vi "Acqusition & Generation (Snapshot) test.vi"() -> ()   [LabVIEW 2014]
uses:
  <vilib>/Platform/TimedLoop/XDataNode/timing_clust.ctl
  <vilib>/Platform/TimedLoop/XDataNode/nitl_modes.ctl
  <vilib>/Platform/TimedLoop/XDataNode/wakeup.ctl
  <vilib>/rvi/Emulation/niFpgaSctlEmulationGetInTimedLoop.vi
  <vilib>/rvi/Emulation/niFpgaEmulationReportErrorSimple.vi
  <vilib>/rvi/Emulation/niFpgaGetClockAttributes.vi
  <vilib>/rvi/Emulation/niFpgaCriticalErrorInLSC.vi
  <vilib>/rvi/Emulation/niFpgaEmulationIsFPGAContextNoSignature.vi
  <vilib>/rvi/DataTransferAndStorage/Container/Common/niFpgaContainerGetUniqueNameForEmu.vi
  <vilib>/rvi/Memory/Memory_Emulation/niFpgaMemoryEmulationCacheClearOnFirstRun.vi
  <vilib>/rvi/Memory/Memory_Emulation/nirvimemoryEmulationManagerCache_MakeExclusive.vi
  <vilib>/rvi/Memory/Memory_Emulation/niFpgaMemoryEmulationValidateCache.vi
  <vilib>/rvi/Memory/Memory_Emulation/nirvimemoryEmulationManagerCache_InsertValue.vi
  <vilib>/Utility/error.llb/Clear Errors.vi
  <vilib>/rvi/Memory/Memory_Emulation/nirvimemoryEmulationManagerCache_ReleaseExclusive.vi
  <vilib>/rvi/Memory/Memory_Emulation/nirvimemoryEmulationManagerCache_GetValue.vi
  <vilib>/rvi/Memory/Memory_Emulation/nirvimemoryEmulationManagerCache_SetValue.vi
  <vilib>/rvi/Emulation/niFpgaProcessEmulError.vi
  <vilib>/rvi/errors/niFpgaSetErrorForExecOnDevCompSimple.vi
  <vilib>/rvi/eio/common/nirviEmuReportErrorAndStop.vi
  <vilib>/rvi/FIFO/Fifo_Resource/nirvififoEmulationSetSize.vi
  <vilib>/rvi/FIFO/Fifo_Resource/nirviFifoEmulationQueueMgr.vi
  <instcachedir>/0/nirviFifoEmulationQueueMgr_E5CAEC123FF24DC58D834DCA3CDAA9B5.lvgen/nirviFifoEmulationQueueMgr_E5CAEC123FF24DC58D834DCA3CDAA9B5_010.vi
  <vilib>/rvi/FIFO/Fifo_Resource/nirvififoEmulationDetermineInputValidOut.vi
  <vilib>/rvi/FIFO/Fifo_Resource/nirvififoEmulationCreateLock.vi
  <vilib>/rvi/FIFO/Fifo_Resource/nirvififoEmulationObtainLock.vi
  <vilib>/rvi/FIFO/Fifo_Resource/nirvififoEmulationReleaseLock.vi
  <vilib>/rvi/occurrence/nirviWaitOnOccurrenceBase.vi
  <vilib>/rvi/errors/nirviReportUnexpectedCaseInternalError.vi
  <vilib>/rvi/errors/nirviReportUnexpectedCaseInternalError (U32).vi
  <vilib>/rvi/Memory/Memory_Emulation/nirvimemoryFastEmulation.vi
  <vilib>/rvi/Memory/Memory_Emulation/nirvimemoryEmulation.vi
  <vilib>/rvi/interface/RandomDataEmulation/niFpgaRandomDataHandleErrors.vi
  <vilib>/rvi/eio/common/nirviEmuTemplateMethod_errors.vi
  <vilib>/Platform/TimedLoop/XDataNode/XDataNode.xnode
  <vilib>/rvi/DataTransferAndStorage/Container/XNode/niFpgaContainer.xnode
  <vilib>/rvi/DataTransferAndStorage/Register/Emulation/niFpgaRegisterEmulation.vi
  <vilib>/rvi/FIFO/Fifo_Resource/nirvififoEmulationWrite.vi
  <vilib>/rvi/interface/RandomDataEmulation/nirviRandomDataFpgaReadWriteTemplate.vi
  <vilib>/rvi/FIFO/Fifo_Resource/nirvififoEmulationRead.vi
  <vilib>/eio/EIOMethodNode/EIOMethodNode.xnode
  <vilib>/Platform/TimedLoop/XDataNode/XDNodeRunTimeDep.lvlib
panel:
  in  "Snapshot":bool
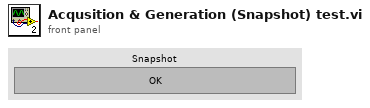
[diagram p1: front panel]
types:
  T1 = typedef "XDNodeRunTimeDep.lvlib/timing_clust.ctl" = cluster{"Expected End [f-1]":u64, "Actual End [f-1]":u64, "Finished Late? [f-1]":bool, "Expected End [i-1]":u64, "Actual End [i-1]":u64, "Finished Late? [i-1]":bool, "Expected Start [i]":u64, "Actual Start [i]":u64, "Expected Start [f]":u64, "Actual Start [f]":u64, "Source Name":string, "Structure Name":string, "Period":i64, "Deadline":i64, "Offset":i64, "Start":i64, "Priority":i32, "Timeout":i32, "Mode":T2, "Wakeup Reason":T3, "Error":errorcluster, "Source Type":string, "Secondary Source Type":string, "Global End Time":u64, "Global Start Time":u64, "Frame Duration":u64, "Iteration Duration":u64, "Assigned CPU":i32, "I/O Scan Engine Mode":u32}
  T2 = typedef "XDNodeRunTimeDep.lvlib/nitl_modes.ctl" = enum32{"No Change", "Process missed periods, maintain original phase", "Discard missed periods, maintain original phase", "Process missed periods, ignore original phase", "Discard missed periods, ignore original phase"}
  T3 = typedef "XDNodeRunTimeDep.lvlib/wakeup.ctl" = enum32{"Normal", "Aborted", "Asynchronous wakeup", "Timing source error", "Timed loop error", "Timeout"}
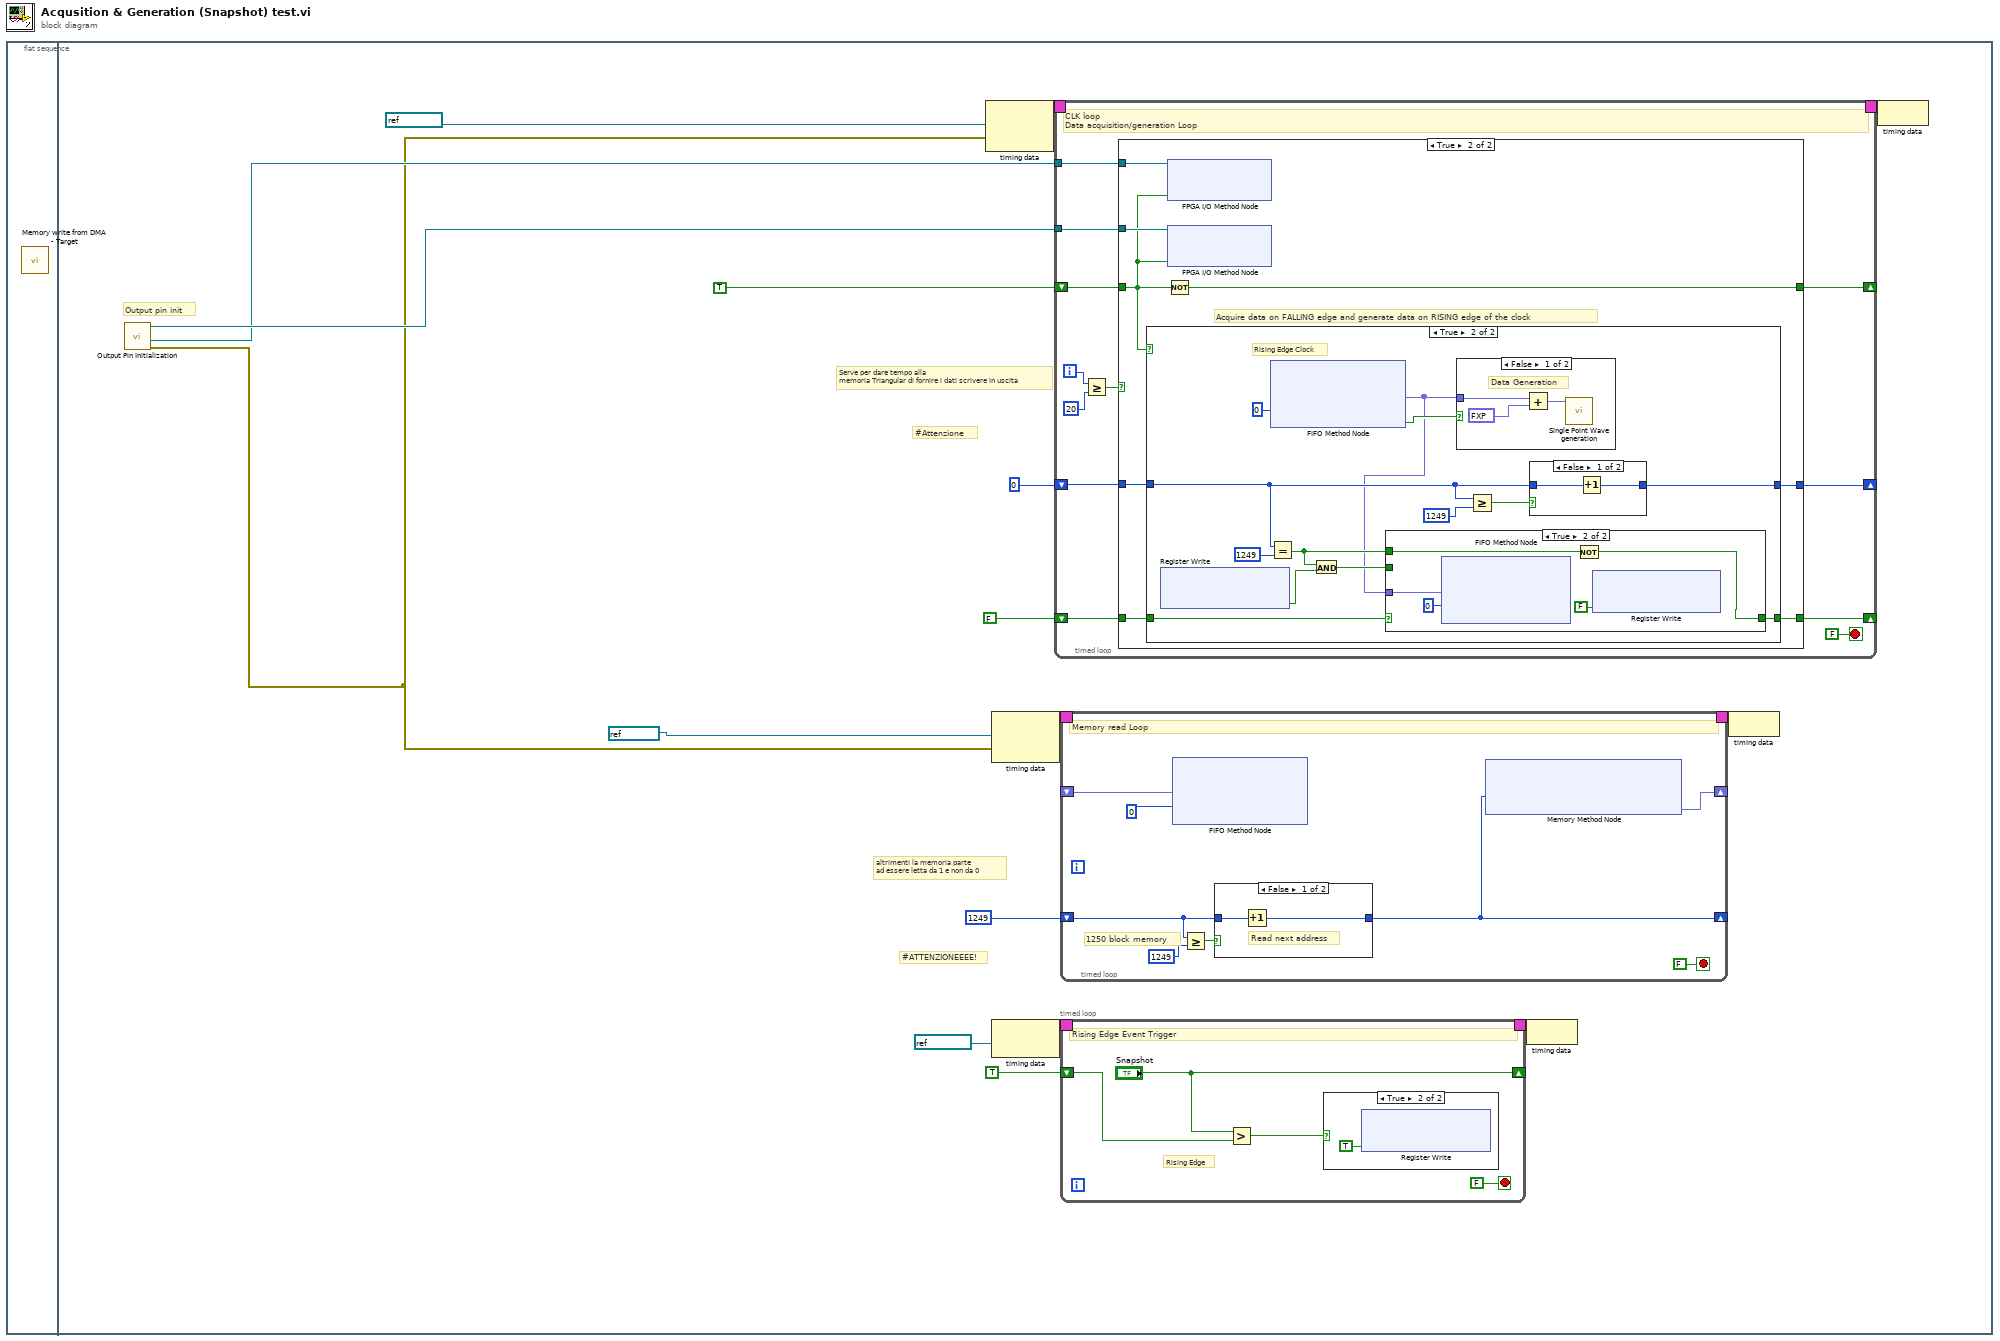
[diagram p0: block diagram]
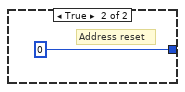
[diagram p3: hidden frame]
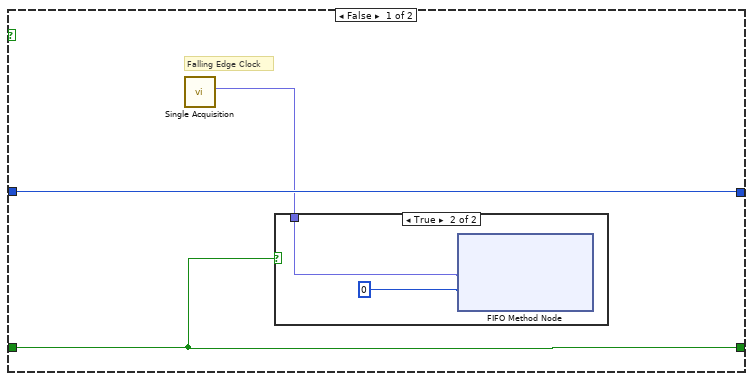
[diagram p5: hidden frame]
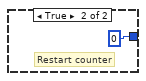
[diagram p9: hidden frame]
diagram:
  n1 = flat-sequence {
    frame #0 {
      n2 = call "Memory write from DMA - Target.vi"() -> ()  [unwired: 12 in]
    }
    frame #1 {
      # "#Attenzione"
      # "Serve per dare tempo alla\nmemoria Triangular di fornire i dati scrivere in uscita"
      # "#ATTENZIONEEEE!"
      # "altrimenti la memoria parte \nad essere letta da 1 e non da 0"
      # "Output pin init"
      n3 = call "Output Pin Initialization.vi"() -> ("error out"=w7:errorcluster, "I/O Out Clock DAC (pin16)"=w8:refnum<k21>, "I/O Out Clock ADC (pin17)"=w9:refnum<k21>)  [unwired: 8 in]
      n4 = node-c288(refnum<k21> "100MHz" ("Source Name"), w7) -> (w17:T1)
      n5 = node-c288(refnum<k21> "50MHz" ("Source Name"), w7) -> (w15:T1)
      n6 = node-c288(refnum<k21> "100MHz" ("Source Name")) -> (w4:T1)
      n7 = timed-loop {
        timing: w17 -> [_]
        timing-out: [_] -> w16
        shift-right: [w56] -> _
        shift-left: TRUE -> [w54]
        tunnel: w8 -> [w58]
        tunnel: w9 -> [w55]
        shift-right: [w53] -> _
        shift-left: i16 0 -> [w52]
        shift-right: [w50] -> _
        shift-left: FALSE -> [w51]
        i -> [w49]
        stop <- FALSE stop-if-true
        # "CLK loop\nData acquisition/generation Loop"
        n8 = Greater Or Equal?(x=w49, y=20) -> (x >= y?=w47:bool)
        n9 = case shown="True" w47 {
          tunnel: w58 -> [_ w69]
          tunnel: [w61 w68] -> w56
          tunnel: w55 -> [_ w67]
          tunnel: w54 -> [w61 w66]
          tunnel: [w60 w65] -> w53
          tunnel: w52 -> [w60 w64]
          tunnel: w51 -> [w59 w63]
          tunnel: [w59 w62] -> w50
          frame False {
          }
          frame True {
            # "Acquire data on FALLING edge and generate data on RISING edge of the clock"
            n10 = case shown="True" w66 {
              tunnel: [w72 w85] -> w65
              tunnel: w64 -> [w72 w80]
              tunnel: w63 -> [w71 w83]
              tunnel: [w71 w81] -> w62
              frame False {
                # "Falling Edge Clock"
                n11 = call "Single Acquisition.vi"() -> ("Out"=w70:fxp<+/-,12,12>)  [unwired: 10 in, 1 out]
                n12 = case shown="True" w71 {
                  tunnel: w70 -> [_ w74]
                  frame False {
                  }
                  frame True {
                    n13 = xnode ("FIFO Method Node")("Element"=w74, "Timeout"=0) -> ()  [unwired: 1 in, 2 out]
                  }
                }
              }
              frame True {
                # "Rising Edge Clock"
                n14 = xnode ("Register Write")() -> ("Data"=w75:bool)  [unwired: 1 in, 1 out]
                n15 = Equal?(x=w80, y=i16 1249) -> (x = y?=w79:bool)
                n16 = xnode ("FIFO Method Node")("Timeout"=0) -> ("Element"=w76:fxp<+/-,12,12>, "Timed Out?"=w77:bool)  [unwired: 1 in, 1 out]
                n17 = And(x=w79, y=w75) -> (x .and. y?=w82:bool)
                n18 = case shown="True" w83 {
                  tunnel: w82 -> [w91 _]
                  tunnel: [w91 w95] -> w81
                  tunnel: w79 -> [_ w96]
                  tunnel: w76 -> [_ w94]
                  frame False {
                  }
                  frame True {
                    n19 = xnode ("FIFO Method Node")("Element"=w94, "Timeout"=0) -> ()  [unwired: 1 in, 2 out]
                    n20 = Not(x=w96) -> (.not. x?=w95:bool)
                    n21 = xnode ("Register Write")("Data"=FALSE) -> ()  [unwired: 1 in, 1 out]
                  }
                }
                n22 = case shown="False" w77 {
                  tunnel: w76 -> [w90 _]
                  frame False {
                    # "Data Generation"
                    n23 = Add(x=w90, y=fxp<+,12,12> 2048.0) -> (x+y=w88:fxp<+/-,14,14>)
                    n24 = call "Single Point Wave generation.vi"("Data To Write"=w88) -> ()  [unwired: 10 in, 1 out]
                  }
                  frame True {
                    # "FPGA memory slow"
                  }
                }
                n25 = Greater Or Equal?(x=w80, y=i16 1249) -> (x >= y?=w86:bool)
                n26 = case shown="False" w86 {
                  tunnel: w80 -> [w98 _]
                  tunnel: [w97 i16 0] -> w85
                  frame False {
                    n27 = Increment(x=w98) -> (x+1=w97:i16)
                  }
                  frame True {
                    # "Restart counter"
                  }
                }
              }
            }
            n28 = Not(x=w66) -> (.not. x?=w68:bool)
            n29 = xnode "FPGA I/O Method Node"("FPGA I/O In"=w69, "Data"=w66) -> ()  [unwired: 1 out]
            n30 = xnode "FPGA I/O Method Node"("FPGA I/O In"=w67, "Data"=w66) -> ()  [unwired: 1 out]
          }
        }
      }
      n31 = timed-loop {
        timing: w15 -> [_]
        timing-out: [_] -> w14
        shift-right: [w29] -> _
        shift-left: u32 1249 -> [w33]
        shift-right: [w31] -> _
        shift-left: _ -> [w30]
        stop <- FALSE stop-if-true
        # "1250 block memory"
        # "Memory read Loop"
        n32 = xnode ("FIFO Method Node")("Element"=w30, "Timeout"=0) -> ()  [unwired: 1 in, 2 out]
        n33 = Greater Or Equal?(x=w33, y=u32 1249) -> (x >= y?=w35:bool)
        n34 = case shown="False" w35 {
          tunnel: w33 -> [w38 _]
          tunnel: [w37 u32 0] -> w29
          frame False {
            # "Read next address"
            n35 = Increment(x=w38) -> (x+1=w37:u32)
          }
          frame True {
            # "Address reset"
          }
        }
        n36 = xnode ("Memory Method Node")("Address"=w29) -> ("Data"=w31:fxp<+/-,12,12>)  [unwired: 1 in, 1 out]
      }
      n37 = timed-loop {
        timing: w4 -> [_]
        timing-out: [_] -> w3
        shift-right: ["Snapshot"] -> _
        shift-left: TRUE ("snapshot") -> [w21]
        stop <- FALSE stop-if-true
        # "Rising Edge"
        # "Rising Edge Event Trigger"
        n38 = Greater?(x="Snapshot", y=w21) -> (0:w19:bool)
        n39 = case shown="True" w19 {
          frame False {
          }
          frame True {
            n40 = xnode ("Register Write")("Data"=TRUE) -> ()  [unwired: 1 in, 1 out]
          }
        }
      }
      n41 = node-c288(w3) -> ()
      n42 = node-c288(w14) -> ()
      n43 = node-c288(w16) -> ()
    }
  }
